vi "Get File Version.vi"(8 "error in (no error)":errorcluster, 11 "Folder Path":path) -> (0 "error out":errorcluster, 3 "File Information":variant)   [LabVIEW 2016, in "File Version Lib.lvlib"]
uses:
  File Version Lib.lvlib
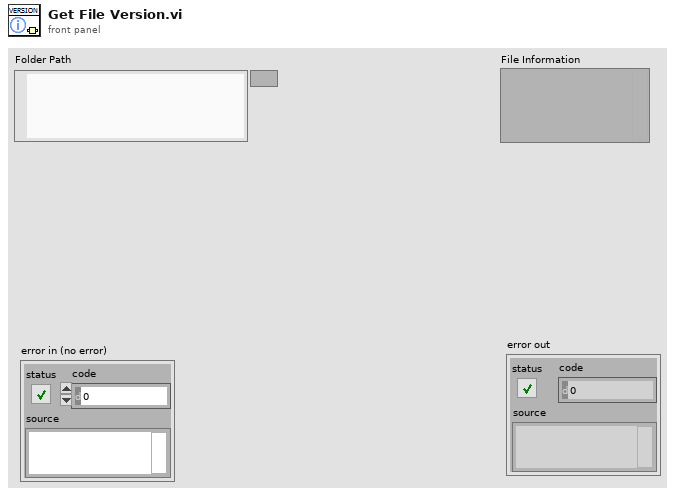
[diagram p1: front panel]
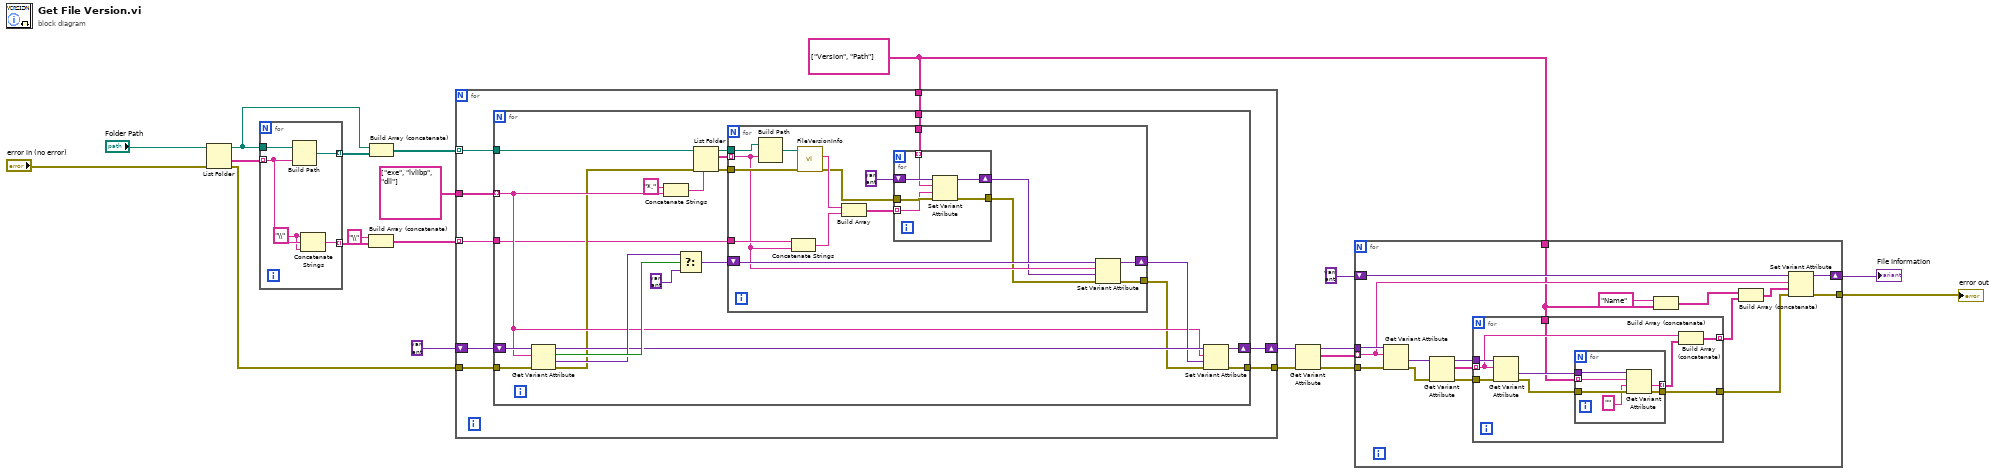
[diagram p0: block diagram]
diagram:
  w2 = string[] ["Version", "Path"]
  n1 = List Folder(path="Folder Path", error in="error in (no error)") -> (path out=w18:path, folder names=w20:string[], error out=w4:errorcluster)  [unwired: 2 in, 1 out]
  n2 = for {
    tunnel: w18 -> [w26]
    tunnel: w20 -> [w24] mode=indexing
    tunnel: [w25] -> w19 mode=indexing
    tunnel: [w23] -> w8 mode=indexing
    w22 = "\\" ("string")
    n3 = Build Path(base path=w26, name or relative path=w24) -> (appended path=w25:path)
    n4 = Concatenate Strings(w22, w24, w22) -> (w23:string)
  }
  n5 = Build Array (concatenate)("\\", w8) -> (w6:string[])
  n6 = Build Array (concatenate)(w18, w19) -> (w17:path[])
  n7 = for {
    tunnel: w17 -> [w34] mode=indexing
    tunnel: string[] ["exe", "lvlibp", "dll"] -> [w33]
    shift-right: [w31] -> w14
    shift-left: variant -> [w32]
    tunnel: [w30] -> w13
    tunnel: w6 -> [w29] mode=indexing
    tunnel: w4 -> [w28]
    tunnel: w2 -> [w27]
    n8 = for {
      tunnel: w34 -> [w55]
      tunnel: w33 -> [w41] mode=indexing
      shift-right: [w43] -> w31
      shift-left: w32 -> [w49]
      tunnel: [w38] -> w30
      tunnel: w29 -> [w37]
      tunnel: w28 -> [w36]
      tunnel: w27 -> [w35]
      n9 = Get Variant Attribute(Variant=w49, name=w41, error in=w36) -> (duplicate Variant=w44:variant, found=w48:bool, value=w47:variant, error out=w40:errorcluster)  [unwired: 1 in]
      n10 = Concatenate Strings("*." ("string"), w41) -> (w54:string)
      n11 = Select(t=w47, s=w48, f=variant) -> (s? t:f=w45:variant)
      n12 = List Folder(path=w55, pattern=w54, error in=w40) -> (path out=w52:path, filenames=w51:string[], error out=w50:errorcluster)  [unwired: 1 in, 1 out]
      n13 = for {
        tunnel: w52 -> [w70]
        tunnel: w51 -> [w64] mode=indexing
        tunnel: w50 -> [w71]
        shift-right: [w67] -> w42
        shift-left: w45 -> [w68]
        tunnel: [w66] -> w39
        tunnel: w37 -> [w65]
        tunnel: w35 -> [w56]
        n14 = Build Path(base path=w70, name or relative path=w64) -> (appended path=w69:path)
        n15 = Concatenate Strings(w65, w64) -> (w63:string)
        n16 = call <vilib>:"FileVersionInfo.vi"("error in (no error)"=w71, "Application Path in"=w69) -> ("error out"=w59:errorcluster, "File Version Info"=w62:string)  [unwired: 6 in, 2 out]
        n17 = Build Array(w62, w63) -> (w61:string[])
        n18 = for {
          tunnel: w61 -> [w75] mode=indexing
          shift-right: [w74] -> w57
          shift-left: variant -> [w77]
          tunnel: w59 -> [w76]
          tunnel: [w73] -> w58
          tunnel: w56 -> [w72] mode=indexing
          n19 = Set Variant Attribute(Variant=w77, name=w72, value=w75, error in=w76) -> (Variant out=w74:variant, error out=w73:errorcluster)  [unwired: 1 out]
        }
        n20 = Set Variant Attribute(Variant=w68, name=w64, value=w57, error in=w58) -> (Variant out=w67:variant, error out=w66:errorcluster)  [unwired: 1 out]
      }
      n21 = Set Variant Attribute(Variant=w44, name=w41, value=w42, error in=w39) -> (Variant out=w43:variant, error out=w38:errorcluster)  [unwired: 1 out]
    }
  }
  n22 = Get Variant Attribute(Variant=w14, error in=w13) -> (duplicate Variant=w12:variant, names=w11:string[], error out=w10:errorcluster)  [unwired: 2 in, 1 out]
  n23 = for {
    tunnel: w12 -> [w94]
    tunnel: w11 -> [w85] mode=indexing
    tunnel: w10 -> [w93]
    shift-right: [w84] -> w1
    shift-left: variant -> [w87]
    tunnel: [w83] -> w3
    tunnel: w2 -> [w80]
    n24 = Get Variant Attribute(Variant=w94, name=w85, error in=w93) -> (value=w92:variant, error out=w91:errorcluster)  [unwired: 1 in, 2 out]
    n25 = Get Variant Attribute(Variant=w92, error in=w91) -> (duplicate Variant=w89:variant, names=w90:string[], error out=w88:errorcluster)  [unwired: 2 in, 1 out]
    n26 = for {
      tunnel: w90 -> [w101] mode=indexing
      tunnel: w89 -> [w102]
      tunnel: w88 -> [w103]
      tunnel: [w99] -> w82 mode=indexing
      tunnel: [w98] -> w86
      tunnel: w80 -> [w95]
      n27 = Get Variant Attribute(Variant=w102, name=w101, error in=w103) -> (value=w97:variant, error out=w96:errorcluster)  [unwired: 1 in, 2 out]
      n28 = for {
        tunnel: w97 -> [w109]
        tunnel: w95 -> [w108] mode=indexing
        tunnel: w96 -> [w107]
        tunnel: [w105] -> w100 mode=indexing
        tunnel: [w104] -> w98
        n29 = Get Variant Attribute(Variant=w109, name=w108, default value (empty Variant)="", error in=w107) -> (value=w105:string, error out=w104:errorcluster)  [unwired: 2 out]
      }
      n30 = Build Array (concatenate)(w101, w100) -> (w99:string[])
    }
    n31 = Build Array (concatenate)("Name", w80) -> (w79:string[])
    n32 = Build Array (concatenate)(w79, w82) -> (w81:string[][])
    n33 = Set Variant Attribute(Variant=w87, name=w85, value=w81, error in=w86) -> (Variant out=w84:variant, error out=w83:errorcluster)  [unwired: 1 out]
  }
  "File Information" <- w1
  "error out" <- w3
